vi "Bounce Window_Add User.vi"(11 "群組：":T1) -> (2 "是否新增":bool, 3 "User Account Data":T2={"帳號 :"="", "權限等級："=enum."開發人員", "建立時間："="", "修改時間："="", "到期時間："="", "狀態："=enum."可使用", "期限："=enum."一天", "密碼："=""})   [LabVIEW 2015]
uses:
  <vilib>/Utility/miscctls.llb/LVPointTypeDef.ctl
panel:
  in  "取消":bool
  in  "狀態：":T3
  in  "期限：":T4=enum."一天"
  in  "確認":bool
  in  "權限等級：":T1
  in  "帳號 ：":string
  # "新增帳號"
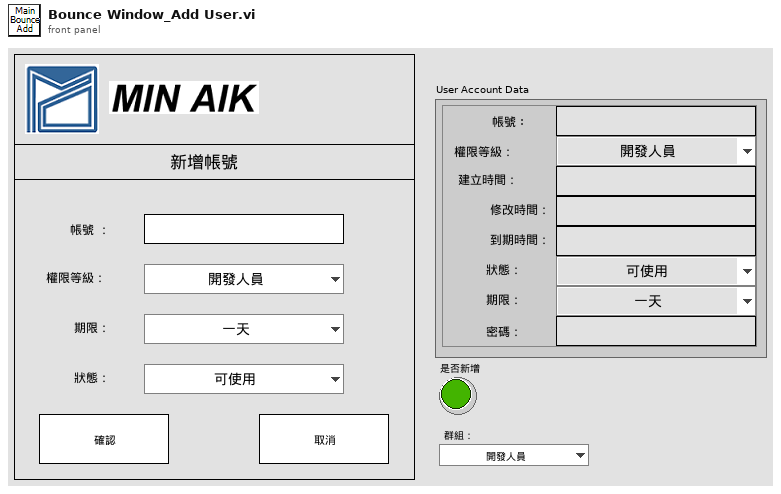
[diagram p1: front panel]
types:
  T1 = typedef "Control_User account_Permissions.ctl" = enum16{"開發人員", "管理者", "工程師", "作業員"}
  T2 = typedef "Control_User account_Data.ctl" = cluster{"帳號 :":string, "權限等級：":T1, "建立時間：":string, "修改時間：":string, "到期時間：":string, "狀態：":T3, "期限：":T4, "密碼：":string}
  T3 = typedef "Control_User Accounts_Status.ctl" = enum16{"可使用", "不可使用"}
  T4 = typedef "Control_User account_Date.ctl" = enum16{"零天", "一天", "七天", "一個月", "一年", "三年"}
  T5 = typedef "LVPointTypeDef.ctl" = cluster{"Horizontal":i16, "Vertical":i16}
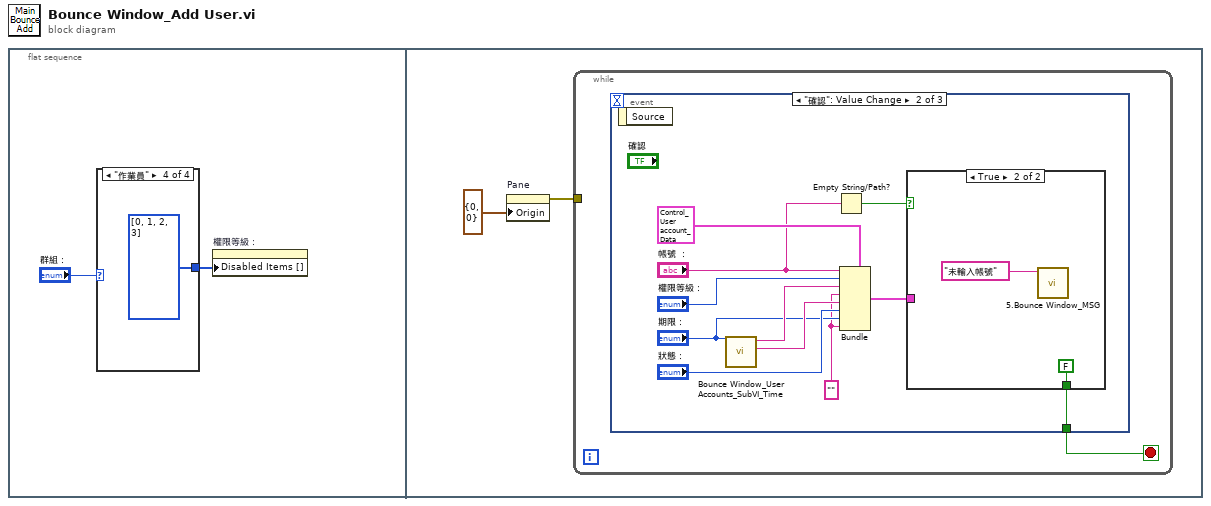
[diagram p0: block diagram]
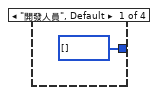
[diagram p2: hidden frame]
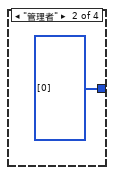
[diagram p3: hidden frame]
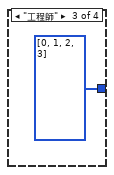
[diagram p4: hidden frame]
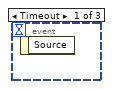
[diagram p5: hidden frame]
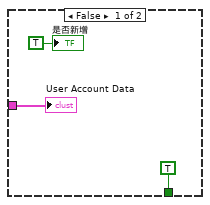
[diagram p6: hidden frame]
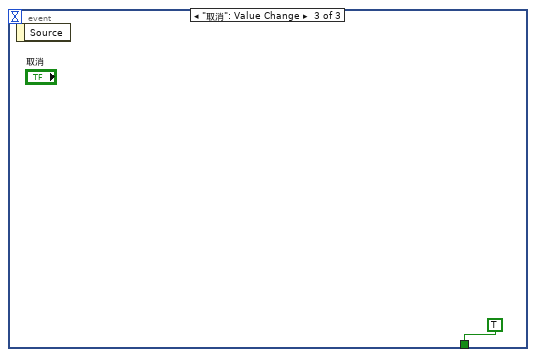
[diagram p7: hidden frame]
diagram:
  n1 = flat-sequence {
    frame #0 {
      n2 = case shown="\"作業員\"" "群組：" {
        tunnel: [i32[] [] ("Disabled Items []") i32[] [0] ("Disabled Items []") i32[] [0, 1, 2, 3] ("Disabled Items []") i32[] [0, 1, 2, 3] ("Disabled Items []")] -> w1
        frame "開發人員", Default {
        }
        frame "管理者" {
        }
        frame "工程師" {
        }
        frame "作業員" {
        }
      }
      n3 = property on="權限等級：" class="Enum (strict)"("Disabled Items []"=w1) -> ()  [unwired: 2 in, 2 out]
    }
    frame #1 {
      n4 = property on="Pane" class="Pane"("Origin"=T5 {"Horizontal"=0, "Vertical"=0}) -> (error out=w7:errorcluster)  [unwired: 2 in, 1 out]
      n5 = while {
        tunnel: w7 -> [_]
        stop <- w9 stop-if-true
        n6 = event shown="[1] \"確認\": Value Change" {
          selector: _ -> [_ _ _]
          dyn-events: _ -> [_ _ _]
          timeout: _ -> [_ _ _]
          tunnel: [_ w10 TRUE] -> w9
          event Timeout {
            n7 = event-data() -> ()  [unwired: 1 in, 1 out]
          }
          event "確認": Value Change {
            w13 = "" ("密碼：")
            n8 = event-data() -> ()  [unwired: 1 in, 1 out]
            n9 = call "Bounce Window_User Accounts_SubVI_Time.vi"("期限："="期限：") -> ("期限"=w17:string, "目前時間"=w18:string)  [unwired: 9 in]
            n10 = Empty String/Path?(string/path="帳號 ：") -> (empty?=w12:bool)
            n11 = Bundle(cluster=T2 {"帳號 :"="", "權限等級："=enum."開發人員", "建立時間："="", "修改時間："="", "到期時間："="", "狀態："=enum."可使用", "期限："=enum."一天", "密碼："=""} ("User Account Data"), "帳號 :"="帳號 ：", "權限等級："="權限等級：", "建立時間："=w18, "修改時間："=w13, "到期時間："=w17, "狀態："="狀態：", "期限："="期限：", "密碼："=w13) -> (w19:T2)
            n12 = case shown="True" w12 {
              tunnel: w19 -> [w23 _]
              tunnel: [TRUE FALSE] -> w10
              frame False {
                "User Account Data" <- w23
                "是否新增" <- TRUE ("是否新增")
              }
              frame True {
                n13 = call "5.Bounce Window_MSG.vi"("MSG In"="未輸入帳號" ("message")) -> ()  [unwired: 11 in]
              }
            }
          }
          event "取消": Value Change {
            n14 = event-data() -> ()  [unwired: 1 in, 1 out]
          }
        }
      }
    }
  }
